vi "Post Message.vi"(6 "Response Timeout(5000ms)":i32=5000, 7 "TcpRouter-Client in":refnum<class "TcpRouter-Client.lvclass">, 8 "error in (no error)":errorcluster, 9 "Target Module":string="Target", 10 "Arguments (\"\")":string, 11 "State":string="API State") -> (0 "error out":errorcluster)   [LabVIEW 2020, in "CSM-TCP-Router.lvlib" / "TcpRouter-Client.lvclass"]
uses:
  TcpRouter-Client.lvclass
  TcpRouter-Client.lvclass/TcpRouter-Client.ctl
  <userlib>/_NEVSTOP/Communicable State Machine(CSM)/Communicable State Machine.lvlib
  _support/tcp-msg type.ctl
  CSM-TCP-Router.lvlib
  ff6050d0-c74c-492c-a255-2017f53df712.vi
  <userlib>/_NEVSTOP/Communicable State Machine(CSM)/_Polymophic/Build Asynchronous Message with Arguments.vi
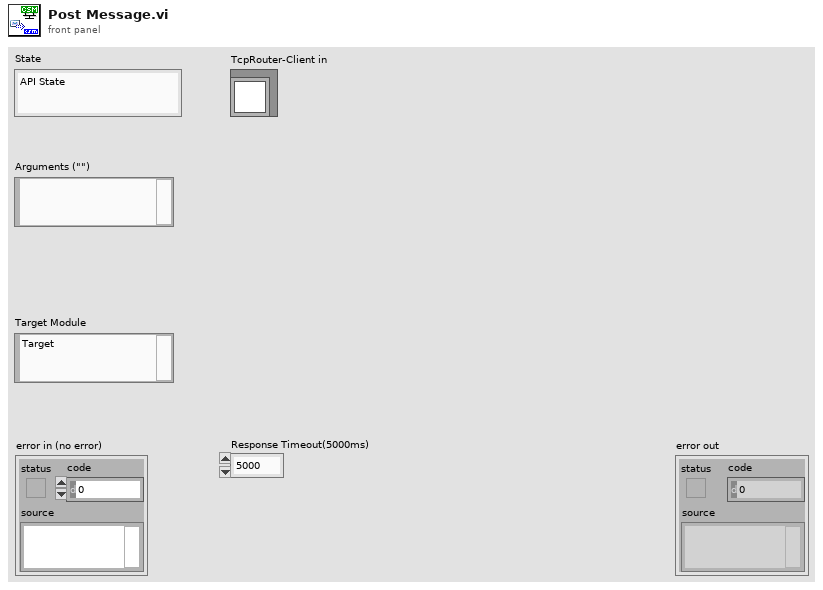
[diagram p1: front panel]
types:
  T1 = typedef "CSM-TCP-Router.lvlib/tcp-msg type.ctl" = enum8{"info", "error", "cmd", "cmd-resp", "resp", "async-resp", "status", "interrupt"}
  T2 = typedef "CSM-TCP-Router.lvlib/TcpRouter-Client.lvclass/Def-TCP-Router ASYNC-RESP.ctl" = cluster{"Async-Resp":refnum<k5>, "RespQueue":refnum<queue>, "RespEvent":refnum<user-event>}
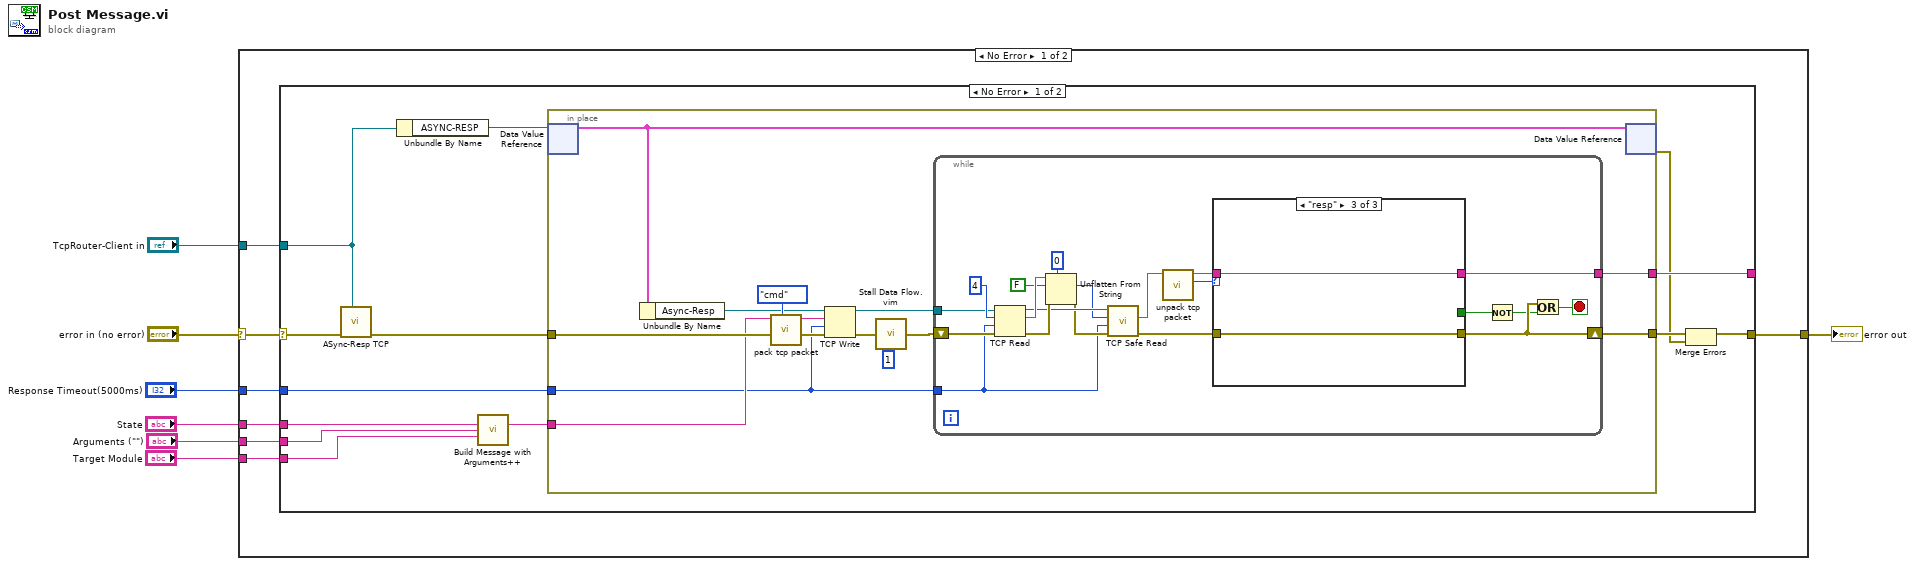
[diagram p0: block diagram]
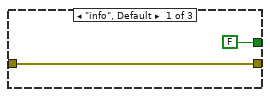
[diagram p2: hidden frame]
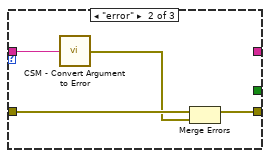
[diagram p3: hidden frame]
diagram:
  n1 = case shown="No Error" "error in (no error)" {
    selector: "error in (no error)" -> [w14 w70]
    tunnel: [w13 w70] -> w6
    tunnel: "TcpRouter-Client in" -> [w12 _]
    tunnel: "Response Timeout(5000ms)" -> [w11 _]
    tunnel: "State" -> [w10 _]
    tunnel: "Arguments (\"\")" -> [w9 _]
    tunnel: "Target Module" -> [w8 _]
    frame No Error {
      n2 = case shown="No Error" w14 {
        selector: w14 -> [w27 w69]
        tunnel: [w18 w69] -> w13
        tunnel: w12 -> [w16 _]
        tunnel: w11 -> [w19 _]
        tunnel: w10 -> [w25 _]
        tunnel: w9 -> [w24 _]
        tunnel: w8 -> [w23 _]
        tunnel: [w20 _] -> _
        frame No Error {
          n3 = call "ASync-Resp TCP.vi"("TcpRouter-Client in"=w16, "error in (no error)"=w27) -> ("error out"=w26:errorcluster)  [unwired: 8 in, 1 out]
          n4 = Unbundle By Name(w16) -> ("ASYNC-RESP"=w15:refnum<data-value>)
          n5 = call-poly <userlib>:"Build Message with Arguments++.vi"("State with Arguments"=w25, "Arguments (\"\")"=w24, "Target Module (\"\")"=w23) -> ("CSM Message String"=w22:string)  [unwired: 12 in]
          n6 = in-place {
            in-place-border: w26 -> [w38]
            in-place-border: w22 -> [w37]
            in-place-border: [w32] -> w21
            in-place-border: [w31] -> w20
            in-place-border: w19 -> [w30]
            n7 = in-place-dvr #1(w15) -> (w29:T2)  [unwired: 1 out]
            n8 = Unbundle By Name(w29) -> ("Async-Resp"=w28:refnum<k5>)
            n9 = call "pack tcp packet.vi"("tcp-message-type"=tcp-msg_type."cmd", "String"=w37) -> ("TCP Pack"=w40:string)  [unwired: 9 in]
            n10 = TCP Write(connection ID=w28, data in=w40, error in (no error)=w38, 9:w30) -> (connection ID out=w34:refnum<k5>, error out=w36:errorcluster)  [unwired: 1 out]
            n11 = call "Stall Data Flow.vim"("value in"=w36, "milliseconds to wait"=u32 1) -> ("value out"=w33:errorcluster)  [unwired: 1 out]
            n12 = while {
              tunnel: w34 -> [w51]
              tunnel: [w46] -> w31
              shift-right: [w45] -> w32
              shift-left: w33 -> [w50]
              tunnel: w30 -> [w44]
              stop <- w43 stop-if-true
              n13 = TCP Read(connection ID=w51, bytes to read=4, error in (no error)=w50, 9:w44) -> (connection ID out=w58:refnum<k5>, data out=w59:string, error out=w60:errorcluster)  [unwired: 1 in]
              n14 = Unflatten From String(type=0, binary string=w59, data includes array or string size? (T)=FALSE, error in (no error)=w60) -> (value=w56:i32, error out=w55:errorcluster)  [unwired: 2 out]
              n15 = call "TCP Safe Read.vi"("error in (no error)"=w55, "timeout ms (25000)"=w44, "bytes to read"=w56, "TCP Network Connection in"=w58) -> ("error out"=w48:errorcluster, "String"=w57:string)  [unwired: 5 in, 1 out]
              n16 = call "unpack tcp packet.vi"("TCP Pack"=w57) -> ("tcp-message-type"=w49:T1, "String"=w47:string)  [unwired: 9 in]
              n17 = case shown="\"resp\"" w49 {
                tunnel: w48 -> [w62 w66 w68]
                tunnel: [w62 w64 w68] -> w45
                tunnel: w47 -> [_ w65 w67]
                tunnel: [_ _ w67] -> w46
                tunnel: [FALSE _ _] -> w42
                frame "info", Default {
                }
                frame "error" {
                  n18 = call <userlib>:"CSM - Convert Argument to Error.vi"("Argument"=w65) -> ("error"=w63:errorcluster)  [unwired: 4 in]
                  n19 = Merge Errors(w66, w63) -> (w64:errorcluster)
                }
                frame "resp" {
                }
              }
              n20 = Not(x=w42) -> (.not. x?=w41:bool)
              n21 = Or(x=w45, y=w41) -> (x .or. y?=w43:bool)
            }
            n22 = in-place-dvr #1(w29) -> (w17:errorcluster)  [unwired: 1 out]
          }
          n23 = Merge Errors(w21, w17) -> (w18:errorcluster)
        }
        frame Error {
        }
      }
    }
    frame Error {
    }
  }
  "error out" <- w6
